vi "Construct TCP Server.vi"(10 "Port":u16, 11 "Service Name":string) -> (3 "TCP Server out":refnum<class "TCP Server.lvclass">)   [LabVIEW 2020, in "TCP Server.lvclass"]
uses:
  <vilib>/gpm_packages/@cs/Network-interface/Source/TCP Interface/TCP Server/TCP Server.lvclass
  <vilib>/gpm_packages/@cs/Network-interface/Source/TCP Interface/TCP Server/TCP Server.lvclass/TCP Server.ctl
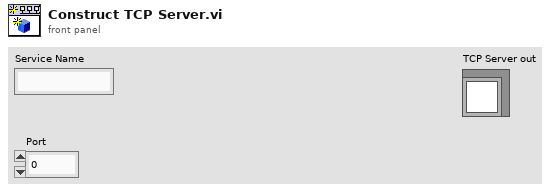
[diagram p1: front panel]
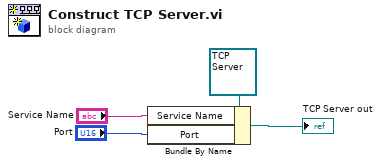
[diagram p0: block diagram]
diagram:
  n1 = Bundle By Name(cluster=refnum<class "TCP Server.lvclass"> refnum ("TCP Server in"), "Service Name"="Service Name", "Port"="Port") -> (→"TCP Server out":refnum<class "TCP Server.lvclass">)
